vi "midiin_main.vi"() -> ()   [LabVIEW 2020]
uses:
  midi/midi.lvclass
panel:
  out "number (0 to 1)":dbl
  out "dwParam2":u32
  out "dwParam1":u32
  out "dwInstance":u32
  out "wMsg":u32
  out "hMidiIn":u32
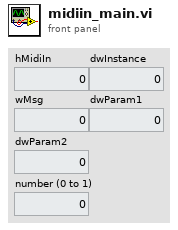
[diagram p1: front panel]
types:
  T1 = cluster{"hMidiIn":u64, "wMsg":u32, "dwInstance":u64, "dwParam1":u64, "dwParam2":u64}
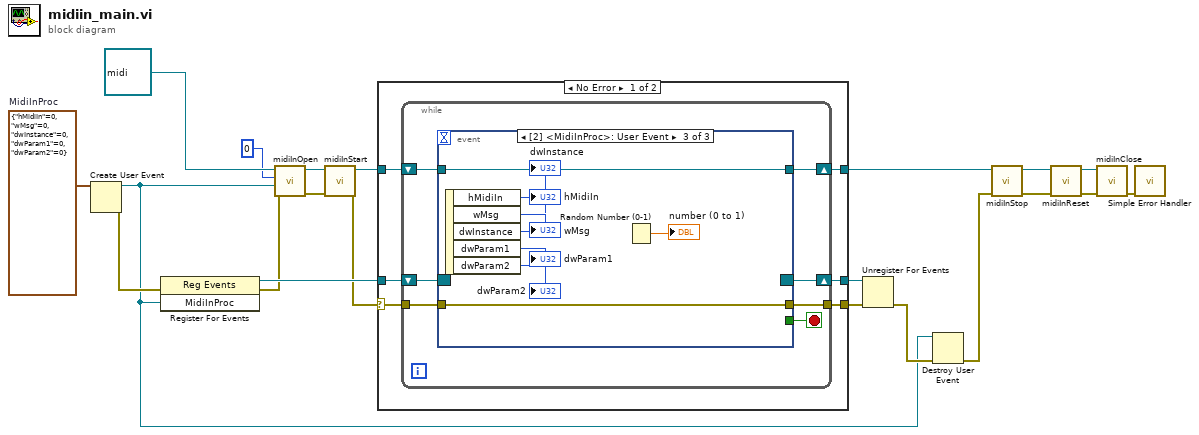
[diagram p0: block diagram]
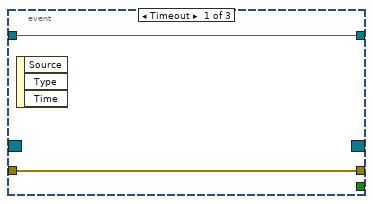
[diagram p2: hidden frame]
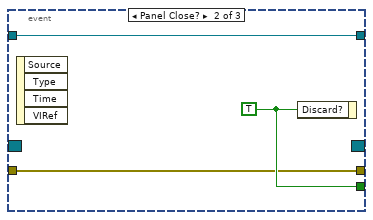
[diagram p3: hidden frame]
diagram:
  w12 = T1 {"hMidiIn"=0, "wMsg"=0, "dwInstance"=0, "dwParam1"=0, "dwParam2"=0}  # MidiInProc
  n1 = Create User Event(user event datatype=w12) -> (user event=w1:refnum<user-event>, error out=w15:errorcluster)  [unwired: 1 in]
  n2 = register-events(error in=w15, w1) -> (reference out=w21:refnum<event-registration>, error out=w17:errorcluster)  [unwired: 1 in]
  n3 = call "midiInOpen.vi"("error in"=w17, "Callback"=w1, "DeviceID"=u32 0, "midi in"=refnum<class "midi.lvclass"> refnum) -> ("error out"=w9:errorcluster, "midi out"=w11:refnum<class "midi.lvclass">)  [unwired: 6 in]
  n4 = call "midiInStart.vi"("error in"=w9, "midi in"=w11) -> ("error out"=w8:errorcluster, "midi out"=w10:refnum<class "midi.lvclass">)  [unwired: 8 in]
  n5 = case shown="No Error" w8 {
    selector: w8 -> [w23 w50]
    tunnel: w21 -> [w27 w49]
    tunnel: [w26 w49] -> w20
    tunnel: w10 -> [w25 w48]
    tunnel: [w24 w50] -> w16
    tunnel: [w22 w48] -> w7
    frame No Error {
      n6 = while {
        shift-right: [w33] -> w26
        shift-left: w27 -> [w34]
        shift-right: [w32] -> w22
        shift-left: w25 -> [w31]
        tunnel: w23 -> [w30]
        tunnel: [w29] -> w24
        stop <- w28 stop-if-true
        n7 = event shown="[2] <MidiInProc>: User Event" {
          selector: w34 -> [_ _ _]
          dyn-events: [_ _ _] -> w33
          timeout: _ -> [_ _ _]
          tunnel: [w36 w39 w47] -> w32
          tunnel: w31 -> [w36 w39 w47]
          tunnel: w30 -> [w35 w37 w46]
          tunnel: [w35 w37 w46] -> w29
          tunnel: [_ w38 _] -> w28
          event Timeout {
            n8 = event-data() -> ()  [unwired: 1 in, 3 out]
          }
          event Panel Close? {
            w38 = TRUE ("Discard?")
            n9 = event-data() -> ()  [unwired: 1 in, 4 out]
            n10 = event-data("Discard?"=w38) -> ()  [unwired: 1 in, 1 out]
          }
          event User Event {
            n11 = event-data() -> ("hMidiIn"=→"hMidiIn":u64, "wMsg"=→"wMsg":u32, "dwInstance"=→"dwInstance":u64, "dwParam1"=→"dwParam1":u64, "dwParam2"=→"dwParam2":u64)  [unwired: 1 in]
            n12 = Random Number (0-1)() -> (number: 0 to 1=→"number (0 to 1)":dbl)
          }
        }
      }
    }
    frame Error {
    }
  }
  n13 = Unregister For Events(event registration refnum=w20, error in=w16) -> (error out=w19:errorcluster)
  n14 = Destroy User Event(user event=w1, error in=w19) -> (error out=w6:errorcluster)
  n15 = call "midiInStop.vi"("error in"=w6, "midi in"=w7) -> ("error out"=w5:errorcluster, "midi out"=w4:refnum<class "midi.lvclass">)  [unwired: 8 in]
  n16 = call "midiInReset.vi"("error in"=w5, "midi in"=w4) -> ("error out"=w3:errorcluster, "midi out"=w2:refnum<class "midi.lvclass">)  [unwired: 8 in]
  n17 = call "midiInClose.vi"("error in"=w3, "midi in"=w2) -> ("error out"=w13:errorcluster)  [unwired: 8 in, 1 out]
  n18 = call <vilib>:"Simple Error Handler.vi"("error in (no error)"=w13) -> ()  [unwired: 4 in, 5 out]
